vi "ToTable.vi"(8 "error in (no error)":errorcluster, 10 "variant":variant, 11 "node in":refnum<class "Shared Memory Editor Node.lvclass">) -> (0 "error out":errorcluster, 2 "table":string[][](array[string]), 3 "node in out":refnum<class "Shared Memory Editor Node.lvclass">)   [LabVIEW 2013, in "Shared Memory Editor Node.lvclass"]
doc: "Copyright 2015 National Instruments Corporation\n\nLicensed under the Apache License, Version 2.0 (the \"License\"); you may not use this file except in compliance with the License. You may obtain a copy of the License at http://www.apache.org/licenses/LICENSE-2.0\nUnless required by applicable law or agreed to in writing, software distributed under the License is distributed on an \"AS IS\" BASIS, WITHOUT WARRANTIES OR CONDITIONS OF ANY KIND, either express or implied. See the License for the specific language governing permissions and limitations under the License."
uses:
  Shared Memory Editor Node.lvclass
  <vilib>/NI/Tag Bus/tag/tag descriptor.lvclass
  <vilib>/NI/Module Execution Interface/Engine Configuration/engine configuration.lvclass
  Shared Memory Editor Node.lvclass/Shared Memory Editor Node.ctl
  module/configuration/Shared Memory Configuration.lvclass/Shared Memory Configuration.ctl
  <vilib>/NI/Configuration Framework/serializable configuration/NISE_CEF_serializable configuration.lvclass/NISE_CEF_serializable configuration.ctl
  <vilib>/NI/Module Execution Interface/Engine Configuration/engine configuration.lvclass/engine configuration.ctl
  <vilib>/NI/Tag Bus Module Framework/channel/TBM channel.lvclass/TBM channel.ctl
  access.ctl
  <vilib>/NI/Tag Bus/tag/tag descriptor.lvclass/tag descriptor.ctl
  module/configuration/Read lines.vi
  <vilib>/Utility/LVClass/Get LV Class Name.vi
  <vilib>/NI/Configuration Framework/error generator/NISE_error generator.vi
  <vilib>/NI/Configuration Framework/serializable configuration/NISE_CEF_serializable configuration.lvclass
  <vilib>/NI/Tag Bus Module Framework/channel/TBM channel.lvclass
  module/configuration/Shared Memory Configuration.lvclass
panel:
  out "tag list":refnum<class "tag descriptor.lvclass">[](array[class])
  out "error out 2":errorcluster
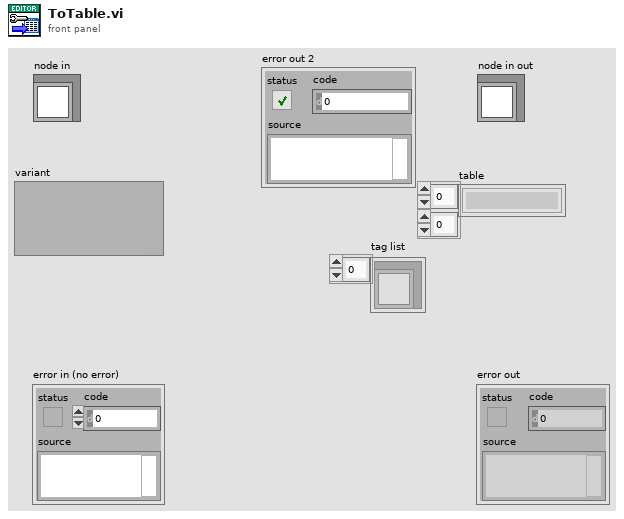
[diagram p1: front panel]
types:
  T1 = typedef "Shared Memory Configuration.lvclass/line configuration.ctl" = cluster{"name":string, "data type":T2, "channel":refnum<class "TBM channel.lvclass">}
  T2 = typedef "tag bus.lvlib/tag descriptor.lvclass/Data Type.ctl" = enum16{"Double", "Single", "I64", "I32", "I16", "I8", "U64", "U32", "U16", "U8", "Boolean", "String", "Array of Double", "Array of Single", "Array of I64", "Array of I32", "Array of I16", "Array of I8", "Array of U64", "Array of U32", "Array of U16", "Array of U8", "Array of Boolean", "Array of String"}
  T3 = typedef "Shared Memory Editor Node.lvclass/access.ctl" = enum16{"Read from File", "Write to File"}
  T4 = typedef "TBM channel.lvclass/channel classification.ctl" = enum16{"input data", "output data", "processing parameter", "processing result"}
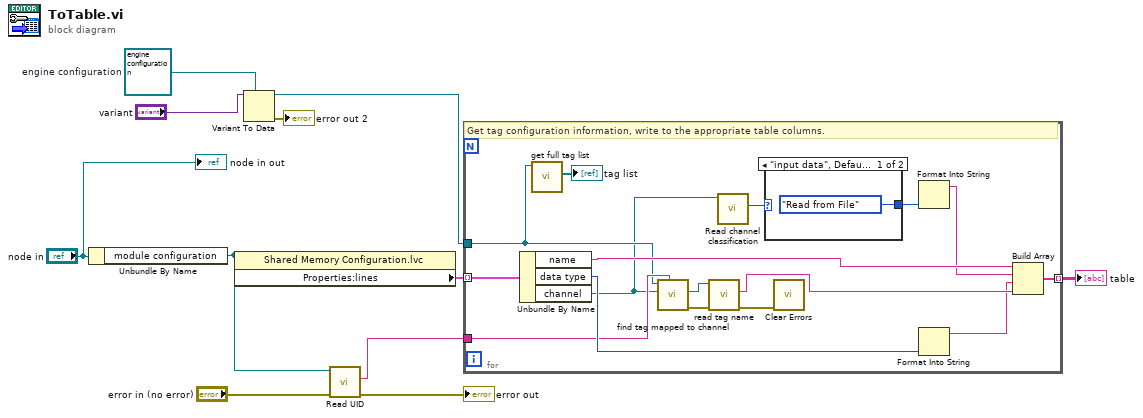
[diagram p0: block diagram]
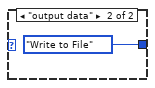
[diagram p2: hidden frame]
diagram:
  w8 = refnum<class "engine configuration.lvclass"> refnum  # engine configuration
  n1 = Unbundle By Name("node in") -> ("module configuration"=w3:refnum<class "Shared Memory Configuration.lvclass">)
  n2 = property class="Shared Memory Configuration.lvc"(reference=w3) -> ("Properties:lines"=w10:T1[])  [unwired: 1 in, 2 out]
  n3 = Variant To Data(type=w8, Variant="variant") -> (data=w9:refnum<class "engine configuration.lvclass">, error out=→"error out 2":errorcluster)  [unwired: 1 in]
  n4 = call <vilib>:"Read UID.vi"("error in"="error in (no error)", "configuration in"=w3) -> ("error out"=→"error out":errorcluster, "instance id"=w11:string)  [unwired: 7 in, 1 out]
  n5 = for {
    tunnel: w10 -> [w27] mode=indexing
    tunnel: w9 -> [w19]
    tunnel: w11 -> [w20]
    tunnel: [w23] -> w7 mode=indexing
    # "Get tag configuration information, write to the appropriate table columns."
    n6 = Unbundle By Name(w27) -> ("name"=w25:string, "data type"=w24:T2, "channel"=w15:refnum<class "TBM channel.lvclass">)
    n7 = call <vilib>:"get full tag list.vi"("engine configuration in"=w19) -> ("tag list"=→"tag list":refnum<class "tag descriptor.lvclass">[])  [unwired: 9 in, 1 out]
    n8 = call <vilib>:"find tag mapped to channel.vi"("owner"=w20, "channel"=w15, "engine configuration in"=w19) -> ("error out"=w22:errorcluster, "tag"=w26:refnum<class "tag descriptor.lvclass">)  [unwired: 6 in, 1 out]
    n9 = call <vilib>:"read tag name.vi"("error in"=w22, "system tag in"=w26) -> ("error out"=w21:errorcluster, "name"=w17:string)  [unwired: 7 in, 1 out]
    n10 = call <vilib>:"Read channel classification.vi"("channel in"=w15) -> ("channel classification"=w14:T4)  [unwired: 8 in, 2 out]
    n11 = case shown="\"input data\", Default" w14 {
      tunnel: [access."Read from File" ("access") access."Write to File" ("access")] -> w12
      frame "input data", Default {
      }
      frame "output data" {
      }
    }
    n12 = call <vilib>:"Clear Errors.vi"("error in (no error)"=w21) -> ()  [unwired: 6 in, 1 out]
    n13 = Format Into String(w12) -> (resulting string=w13:string)  [unwired: 3 in, 1 out]
    n14 = Format Into String(w24) -> (resulting string=w16:string)  [unwired: 3 in, 1 out]
    n15 = Build Array(w25, w13, w16, w17) -> (w23:string[])
  }
  "table" <- w7
  "node in out" <- "node in"
